vi "DBL Array to Result.vi"(7 "Result name":string, 8 "error in (no error)":errorcluster, 10 "Data":dbl[](array[numeric]), 11 "Channel Names":string[](array[string])) -> (0 "error out":errorcluster, 3 "Mag Lab Result out":refnum<class "Mag Lab Result.lvclass">)   [LabVIEW 2015]
uses:
  Mag Lab Result.lvclass
  Waveform Array Result/Waveform Array Result.lvclass
  Mag Lab Result.lvclass/Mag Lab Result.ctl
  Waveform Array Result/Waveform Array Result.lvclass/Waveform Array Result.ctl
  Write Group Name.vi
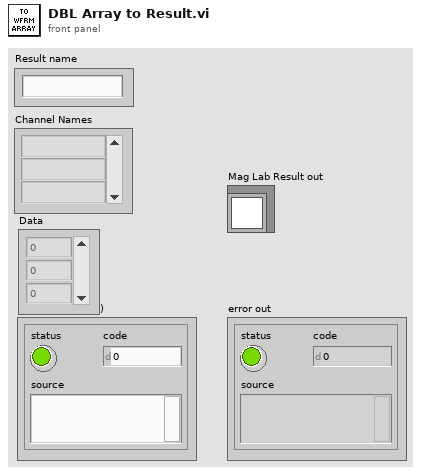
[diagram p1: front panel]
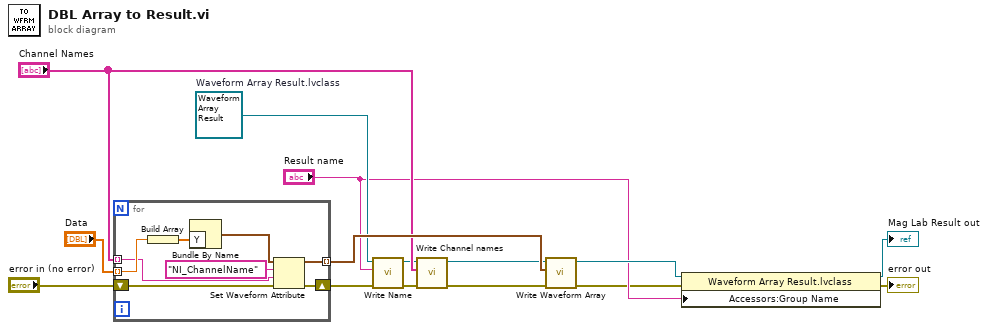
[diagram p0: block diagram]
diagram:
  w6 = refnum<class "Waveform Array Result.lvclass"> refnum  # Waveform Array Result.lvclass
  n1 = for {
    tunnel: "Data" -> [w21] mode=indexing
    tunnel: "Channel Names" -> [w19] mode=indexing
    shift-right: [w17] -> w9
    shift-left: "error in (no error)" -> [w18]
    tunnel: [w16] -> w13 mode=indexing
    n2 = Build Array(w21) -> (w20:dbl[])
    n3 = Bundle By Name("Y"=w20) -> (w22:waveform(dbl))  [unwired: 1 in]
    n4 = Set Waveform Attribute(4:w18, 5:w19, 6:"NI_ChannelName", 7:w22) -> (0:w17:errorcluster, 3:w16:waveform(dbl))  [unwired: 1 out]
  }
  n5 = call "Write Name.vi"("error in (no error)"=w9, "Name"="Result name", "Mag Lab Result in"=w6) -> ("error out"=w8:errorcluster, "Mag Lab Result out"=w7:refnum<class "Waveform Array Result.lvclass">)  [unwired: 7 in]
  n6 = call "Write Channel names.vi"("error in (no error)"=w8, "Channel names"="Channel Names", "Waveform Array Result in"=w7) -> ("error out"=w10:errorcluster, "Waveform Array Result out"=w11:refnum<class "Waveform Array Result.lvclass">)  [unwired: 7 in]
  n7 = call "Write Waveform Array.vi"("error in (no error)"=w10, "Waveform Array"=w13, "Waveform Array Result in"=w11) -> ("error out"=w2:errorcluster, "Waveform Array Result out"=w5:refnum<class "Waveform Array Result.lvclass">)  [unwired: 7 in]
  n8 = property class="Waveform Array Result.lvclass"(reference=w5, error in=w2, "Accessors:Group Name"="Result name") -> (reference out=→"Mag Lab Result out":refnum<class "Waveform Array Result.lvclass">, error out=→"error out":errorcluster)
